vi "Teleop.vi"(10 "Match Info":T1={"Autonomous Elapsed Seconds"=0.0, "TeleOp Elapsed Seconds"=0.0, "Disabled Elapsed Seconds"=0.0, "Visited Autonomous"=FALSE, "Visited TeleOp"=FALSE, "Visited Disabled"=FALSE, "Autonomous Settings"={"Autonomous Style"=enum."Independent", "VI Refnum"=refnum}}, 11 "Call Context":T2) -> ()   [LabVIEW 2015]
doc: "This VI is called for each TeleOp packet received from the DS where the robot is not disabled. It is often used to read from the joysticks and update I/O or to update setpoints for timed control loops. It should complete and return within 20 milliseconds or it may miss DS packets."
uses:
  <vilib>/Rock Robotics/WPI/DriverStation/WPI_DriverStationDerivedRobotMode.ctl
  <vilib>/Rock Robotics/WPI/DriverStation/WPI_DriverStationMatch Info.ctl
  <vilib>/Rock Robotics/Network Tables/NT Read Boolean.vi
  <vilib>/Rock Robotics/Network Tables/NT Read Number.vi
  <vilib>/Rock Robotics/WPI/Utilities/WPI_GetSetVariantRefNum.vi
  Team Code/Global_Var/JoyStick_Global.vi
panel:
  out "Sample Slider 0":dbl(slide) scale=0.0..5.0
  out "Sample Boolean 1":bool
  out "Sample Boolean 0":bool
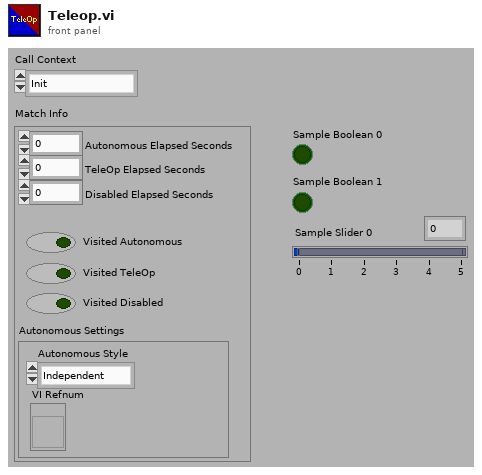
[diagram p1: front panel]
types:
  T1 = typedef "WPI_DriverStationMatch Info.ctl" = cluster{"Autonomous Elapsed Seconds":dbl, "TeleOp Elapsed Seconds":dbl, "Disabled Elapsed Seconds":dbl, "Visited Autonomous":bool, "Visited TeleOp":bool, "Visited Disabled":bool, "Autonomous Settings":cluster{"Autonomous Style":enum16{"Iterative", "Independent"}, "VI Refnum":refnum<vi>}}
  T2 = typedef "WPI_DriverStationDerivedRobotMode.ctl" = enum16{"Init", "Execute", "Stop"}
  T3 = typedef "WPI_JoystickDevRef.ctl" = cluster{"Device":T4}
  T4 = typedef "WPI_JoystickDeviceEnum.ctl" = enum16{"USB 0", "USB 1", "USB 2", "USB 3", "USB 4", "USB 5"}
  T5 = cluster{"Left_Trigger":dbl, "Right_Trigger ":dbl, "Left_X":dbl, "Left_Y":dbl, "Right_X":dbl, "Right_Y":dbl}
  T6 = cluster{"A":bool, "B":bool, "X":bool, " Y":bool, "LB":bool, " RB":bool, "Left_Thumb_Button":bool, "Right_Thumb_Button":bool, "Back":bool, "Start":bool}
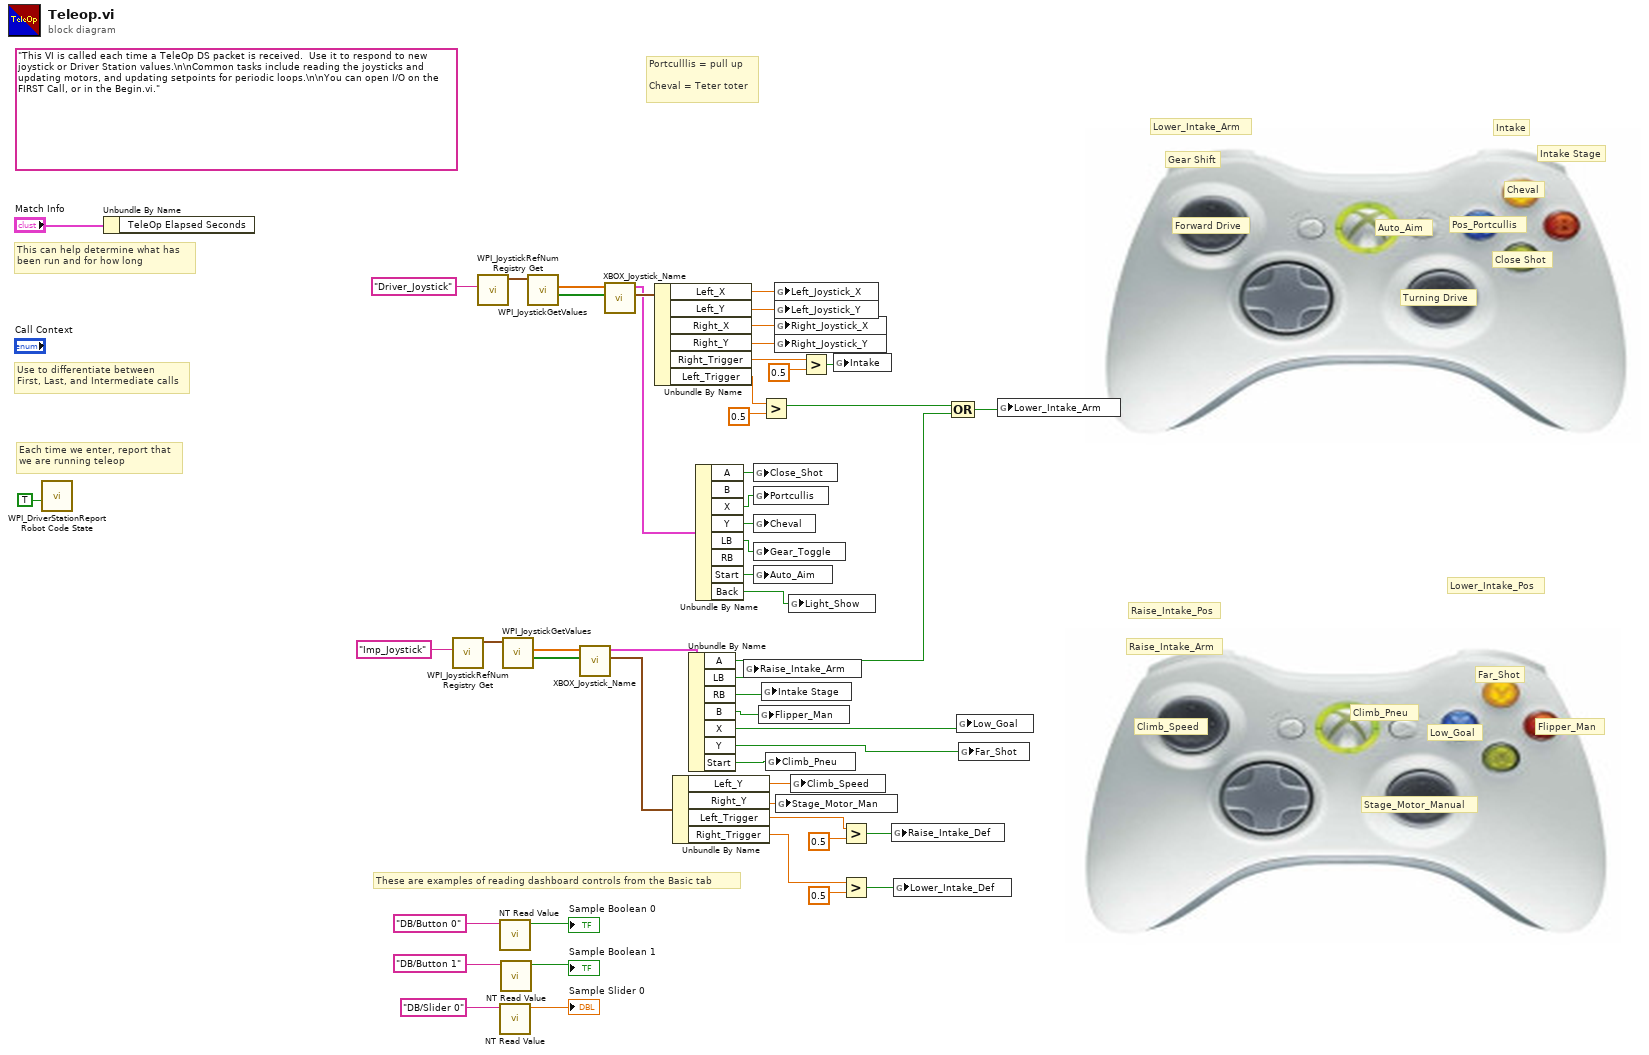
[diagram p0: block diagram]
diagram:
  (unwired) "This VI is called each time a TeleOp DS packet is received.  Use it to respond to new joystick or Driver Station values.\n\nCommon tasks include reading the joysticks and updating motors, and updating setpoints for periodic loops.\n\nYou can open I/O on the FIRST Call, or in the Begin.vi."
  # "Low_Goal"
  # "Climb_Pneu"
  # "Auto_Aim"
  # "Intake"
  # "Flipper_Man"
  # "Lower_Intake_Pos"
  # "Raise_Intake_Pos"
  # "Lower_Intake_Arm"
  # "Raise_Intake_Arm"
  # "Stage_Motor_Manual"
  # "Climb_Speed"
  # "Intake Stage"
  # "Gear Shift"
  # "Cheval"
  # "Portculllis = pull up\n\nCheval = Teter toter"
  # "Pos_Portcullis"
  # "Far_Shot"
  # "Close Shot"
  # "Turning Drive"
  # "Forward Drive"
  # "These are examples of reading dashboard controls from the Basic tab"
  # "Each time we enter, report that\nwe are running teleop"
  # "Use to differentiate between\nFirst, Last, and Intermediate calls"
  # "This can help determine what has\nbeen run and for how long"
  n1 = call <vilib>:"WPI_DriverStationReport Robot Code State.vi"("TeleOp"=TRUE ("Autonomous")) -> ()  [unwired: 10 in, 1 out]
  n2 = Unbundle By Name("Match Info") -> ()  [unwired: 1 out]
  n3 = call <vilib>:"WPI_JoystickRefNum Registry Get.vi"("refnum name"="Imp_Joystick") -> ("JoystickDevRef"=w41:T3)  [unwired: 1 in, 9 out]
  n4 = call <vilib>:"WPI_JoystickRefNum Registry Get.vi"("refnum name"="Driver_Joystick") -> ("JoystickDevRef"=w51:T3)  [unwired: 1 in, 9 out]
  n5 = call-poly <vilib>:"NT Read Value.vi"("Name"="DB/Button 0" ("refnum name")) -> ("Boolean"=→"Sample Boolean 0":bool)  [unwired: 9 in, 1 out]
  n6 = call-poly <vilib>:"NT Read Value.vi"("Name"="DB/Slider 0" ("refnum name")) -> ("Numeric"=→"Sample Slider 0":dbl)  [unwired: 9 in, 1 out]
  n7 = call-poly <vilib>:"NT Read Value.vi"("Name"="DB/Button 1" ("refnum name")) -> ("Boolean"=→"Sample Boolean 1":bool)  [unwired: 9 in, 1 out]
  n8 = call <vilib>:"WPI_JoystickGetValues.vi"("JoystickDevRef"=w41) -> ("Buttons"=w39:bool[], "Axes"=w40:dbl[])  [unwired: 6 in, 3 out]
  n9 = call <vilib>:"WPI_JoystickGetValues.vi"("JoystickDevRef"=w51) -> ("Buttons"=w42:bool[], "Axes"=w43:dbl[])  [unwired: 6 in, 3 out]
  n10 = call "XBOX_Joystick_Name.vi"("Buttons"=w39, "Axes"=w40) -> ("Named_Joystick"=w22:T5, "Named_Buttons"=w23:T6)  [unwired: 8 in]
  n11 = call "XBOX_Joystick_Name.vi"("Buttons"=w42, "Axes"=w43) -> ("Named_Joystick"=w36:T5, "Named_Buttons"=w29:T6)  [unwired: 8 in]
  n12 = Unbundle By Name(w36) -> ("Left_X"=w35:dbl, "Left_Y"=w34:dbl, "Right_X"=w33:dbl, "Right_Y"=w32:dbl, "Right_Trigger"=w26:dbl, "Left_Trigger"=w11:dbl)
  n13 = Unbundle By Name(w22) -> ("Left_Y"=w5:dbl, "Right_Y"=w21:dbl, "Left_Trigger"=w18:dbl, "Right_Trigger"=w16:dbl)
  n14 = Unbundle By Name(w23) -> ("A"=w6:bool, "LB"=w20:bool, "RB"=w9:bool, "B"=w13:bool, "X"=w2:bool, "Y"=w4:bool, "Start"=w3:bool)
  n15 = Unbundle By Name(w29) -> ("A"=w31:bool, "X"=w30:bool, "Y"=w28:bool, "LB"=w27:bool, "Start"=w10:bool, "Back"=w1:bool)  [unwired: 2 out]
  n16 = global write "JoyStick_Global.vi" "Raise_Intake_Arm"(w20) -> ()
  n17 = global write "JoyStick_Global.vi" "Close_Shot"(w31) -> ()
  n18 = global write "JoyStick_Global.vi" "Portcullis"(w30) -> ()
  n19 = global write "JoyStick_Global.vi" "Cheval"(w28) -> ()
  n20 = global write "JoyStick_Global.vi" "Gear_Toggle"(w27) -> ()
  n21 = global write "JoyStick_Global.vi" "Auto_Aim"(w10) -> ()
  n22 = global write "JoyStick_Global.vi" "Flipper_Man"(w13) -> ()
  n23 = Greater?(x=w11, y=0.5) -> (0:w8:bool)
  n24 = global write "JoyStick_Global.vi" "Intake Stage"(w9) -> ()
  n25 = global write "JoyStick_Global.vi" "Climb_Pneu"(w3) -> ()
  n26 = global write "JoyStick_Global.vi" "Left_Joystick_X"(w35) -> ()
  n27 = global write "JoyStick_Global.vi" "Left_Joystick_Y"(w34) -> ()
  n28 = global write "JoyStick_Global.vi" "Right_Joystick_X"(w33) -> ()
  n29 = global write "JoyStick_Global.vi" "Right_Joystick_Y"(w32) -> ()
  n30 = global write "JoyStick_Global.vi" "Stage_Motor_Man"(w21) -> ()
  n31 = global write "JoyStick_Global.vi" "Light_Show"(w1) -> ()
  n32 = global write "JoyStick_Global.vi" "Climb_Speed"(w5) -> ()
  n33 = Greater?(x=w26, y=0.5) -> (0:w24:bool)
  n34 = global write "JoyStick_Global.vi" "Intake"(w24) -> ()
  n35 = Greater?(x=w18, y=0.5) -> (0:w14:bool)
  n36 = Greater?(x=w16, y=0.5) -> (0:w15:bool)
  n37 = global write "JoyStick_Global.vi" "Raise_Intake_Def"(w14) -> ()
  n38 = global write "JoyStick_Global.vi" "Lower_Intake_Def"(w15) -> ()
  n39 = Compound Arithmetic op=OR(w8, w6) -> (w7:bool)
  n40 = global write "JoyStick_Global.vi" "Low_Goal"(w2) -> ()
  n41 = global write "JoyStick_Global.vi" "Far_Shot"(w4) -> ()
  n42 = global write "JoyStick_Global.vi" "Lower_Intake_Arm"(w7) -> ()
